vi "add_bool.vi"   [LabVIEW 2010]
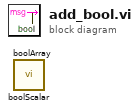
[diagram p0: block diagram]
diagram:
  n1 = call <userlib>:"boolScalar.vi"() -> ()  [unwired: 5 in, 1 out]
  n2 = call <userlib>:"boolArray.vi"() -> ()  [unwired: 5 in, 1 out]
